vi "To Binary.vi"(8 "error in (no error)":errorcluster, 9 "byte order":T1(ring), 10 "Binary In":string, 11 "Double Float in":refnum<class "AbsFunc_Two Term_DBL.lvclass">) -> (0 "error out":errorcluster, 2 "Binary":string, 3 "Double Float out":refnum<class "AbsFunc_Two Term_DBL.lvclass">)   [LabVIEW 2021, in "AbsFunc_Two Term_DBL.lvclass"]
uses:
  AbsFunc_Two Term_DBL.lvclass
  AbsFunc_Two Term_DBL.lvclass/AbsFunc_Two Term_DBL.ctl
  Abs_Types/Double Float/Abs_Double Float.lvclass
  Abs_Types/Numeric/Abs_Numeric.lvclass
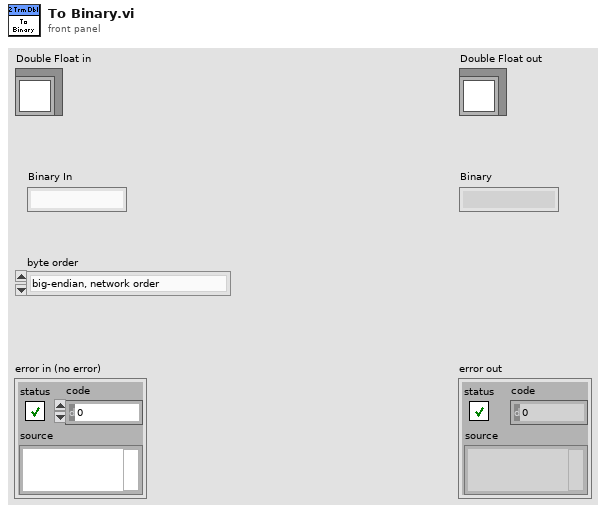
[diagram p1: front panel]
types:
  T1 = enum16{"big-endian, network order", "native, host order", "little-endian"}
  T2 = typedef "AbsFunc_Two Term DBL.lvclass/Abstract Type.ctl" = refnum<class "Abs_Double Float.lvclass">
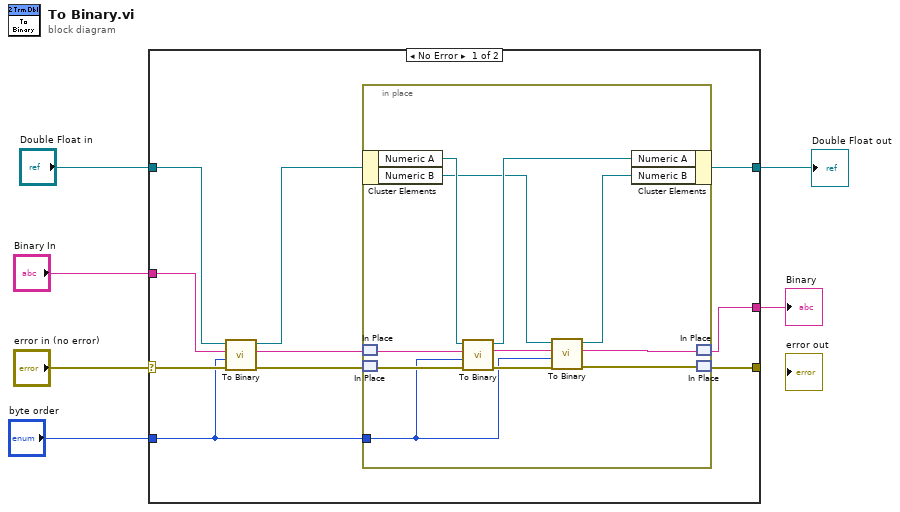
[diagram p0: block diagram]
diagram:
  n1 = case shown="No Error" "error in (no error)" {
    selector: "error in (no error)" -> [w13 w28]
    tunnel: "Binary In" -> [w9 w29]
    tunnel: "Double Float in" -> [w11 w30]
    tunnel: "byte order" -> [w8 _]
    tunnel: [w16 w28] -> _
    tunnel: [w15 w29] -> w1
    tunnel: [w14 w30] -> w2
    frame No Error {
      n2 = call-parent "To Binary.vi"("error in (no error)"=w13, "byte order"=w8, "Binary In"=w9, "Double Float in"=w11) -> ("error out"=w12:errorcluster, "Binary"=w7:string, "Double Float out"=w10:refnum<class "AbsFunc_Two Term_DBL.lvclass">)  [unwired: 5 in]
      n3 = in-place {
        in-place-border: w8 -> [w20]
        n4 = in-place-cluster #1(w10) -> ("Numeric A"=w27:T2, "Numeric B"=w23:refnum<class "Abs_Numeric.lvclass">)
        n5 = in-place-match #2(w7) -> (w25:string)
        n6 = in-place-match #3(w12) -> (w24:errorcluster)
        n7 = call-dynamic "To Binary.vi"("error in (no error)"=w24, "byte order"=w20, "Binary In"=w25, "Double Float in"=w27) -> ("error out"=w22:errorcluster, "Binary"=w21:string, "Double Float out"=w26:T2)  [unwired: 5 in]
        n8 = call-dynamic "To Binary.vi"("error in (no error)"=w22, "byte order"=w20, "Binary In"=w21, "Type in"=w23) -> ("error out"=w17:errorcluster, "Binary"=w18:string, "Type out"=w19:refnum<class "Abs_Numeric.lvclass">)  [unwired: 5 in]
        n9 = in-place-cluster #1("Numeric A"=w26, "Numeric B"=w19) -> (w14:refnum<class "AbsFunc_Two Term_DBL.lvclass">)
        n10 = in-place-match #2(w18) -> (w15:string)
        n11 = in-place-match #3(w17) -> (w16:errorcluster)
      }
    }
    frame Error {
    }
  }
  "Double Float out" <- w2
  "Binary" <- w1
